vi "CRYDataView Close Panel.vi"(8 "Panel_Idx":i32, 11 "DataView Index":i32) -> (0 "bResult":bool, 2 "bHaveChild":bool, 3 "closed_spliter_idx":i32)   [LabVIEW 2013]
uses:
  CRYNew View Global.vi
panel:
  in  "sp_mdown_hei":i32
  in  "sp_mdown_wid":i32
  in  "sp_mdown_ypos":i32
  in  "sp_mdown_xpos":i32
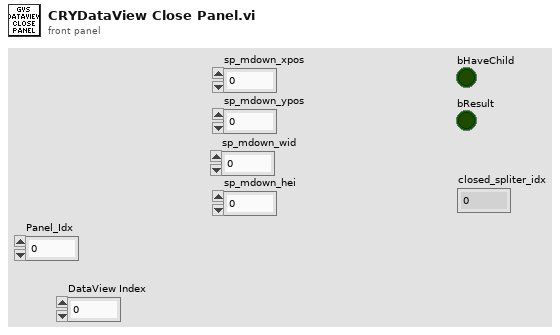
[diagram p1: front panel]
types:
  T1 = typedef "Graph Main Info Cluster.ctl" = cluster{"Selected_BarIdx":i32, "Selected_PanelIdx":i32, "Graph Main VIRef":refnum<vi>, "ToolBarClick":bool, "Spliter Ref Array":refnum<vi>[], "Panel Ref Array":refnum<vi>[], "Spliter_matrix":i32[][], "Panel_matrix":i32[][], "child_spliterIdx_matrix":i32[][], "split_pos_matrix":i32[][], "Title State":bool, "sQueueName":string, "Frame nID":i32, "Graph VIRef Array":cluster{"Graph VIRef":refnum<vi>, "Panel Idx":i32, "Frame VIRef":refnum<vi>, "Icon Ring":i32, "Graph Type":string}[], "View Type":string}
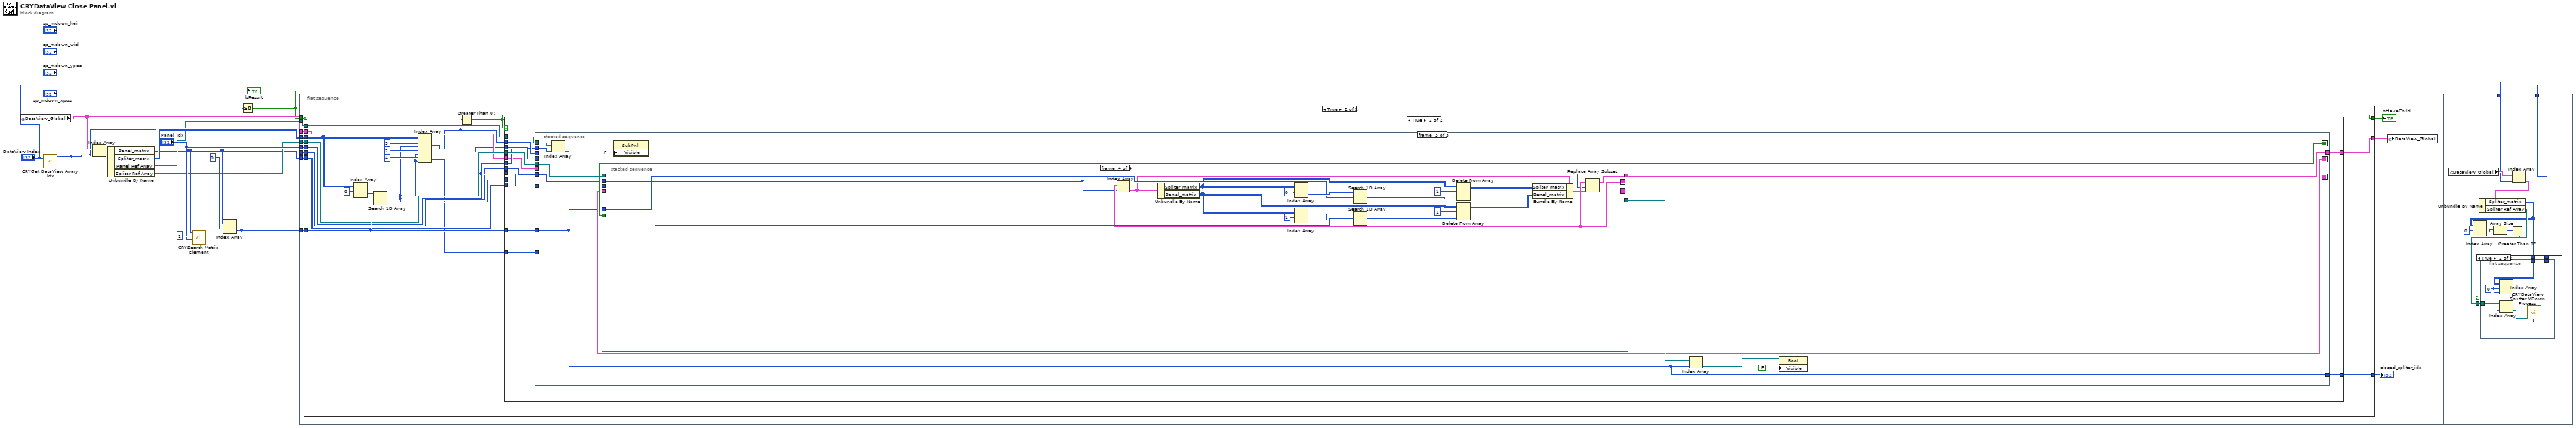
[diagram p0: block diagram]
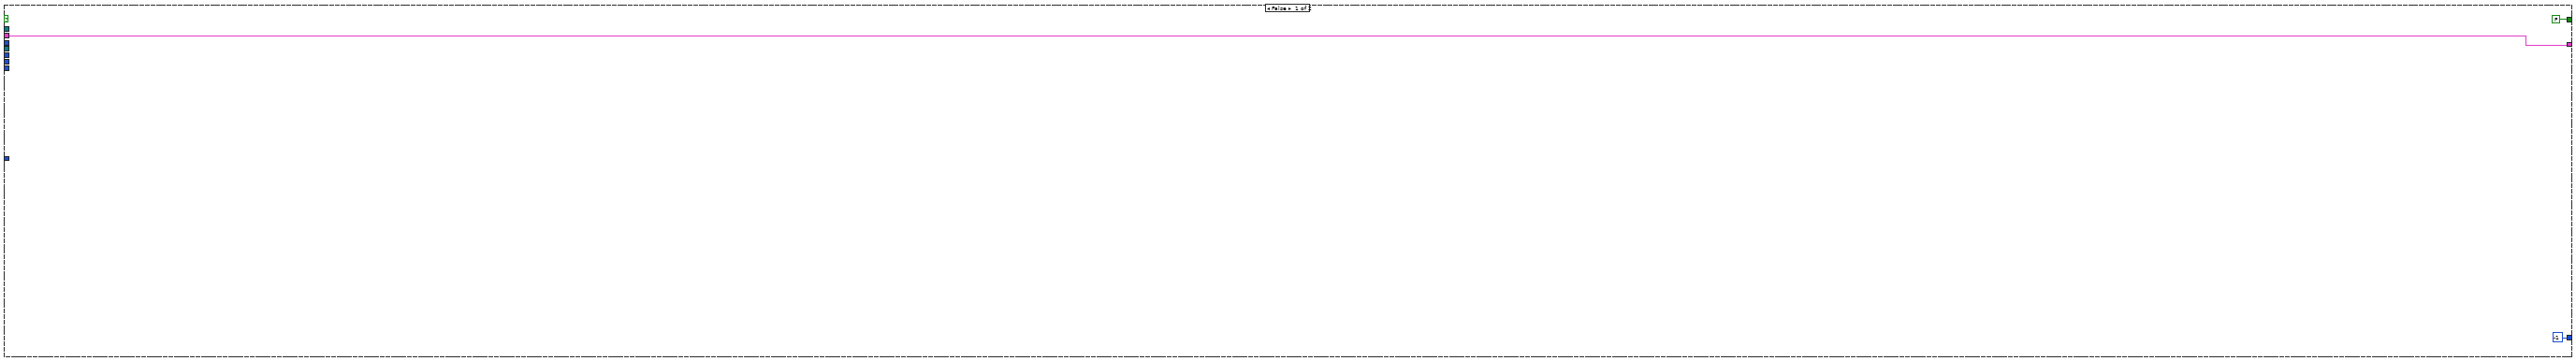
[diagram p2: hidden frame]
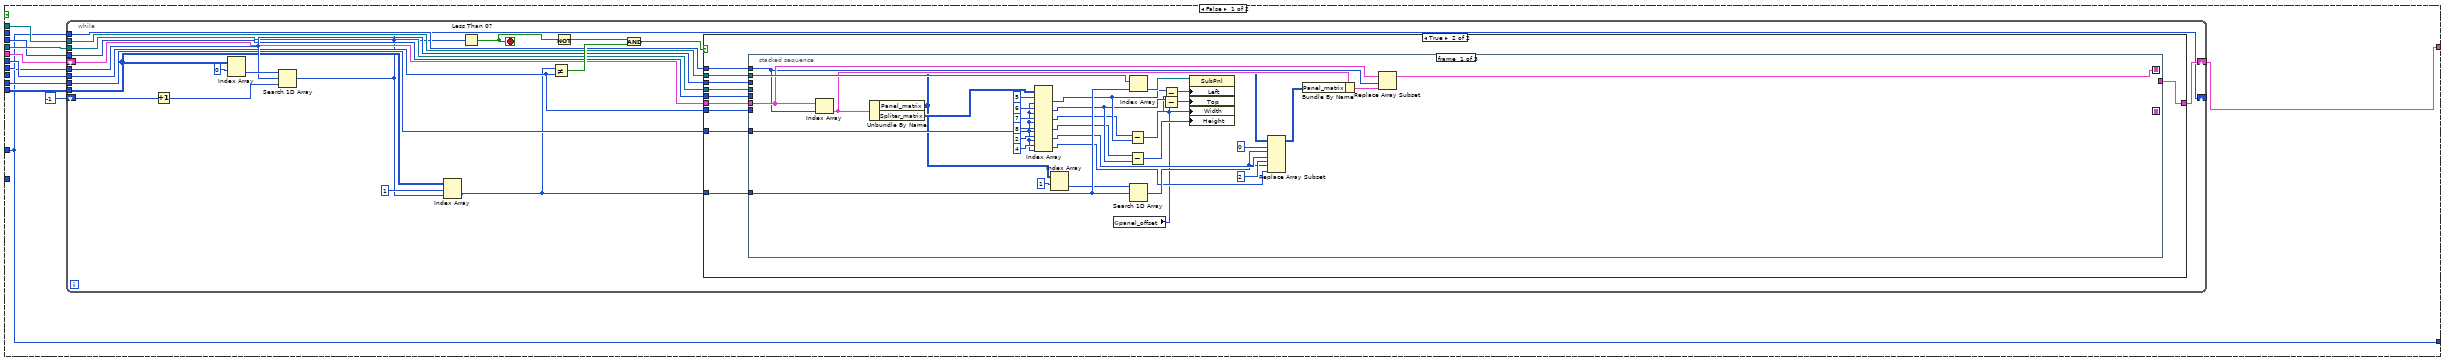
[diagram p3: hidden frame]
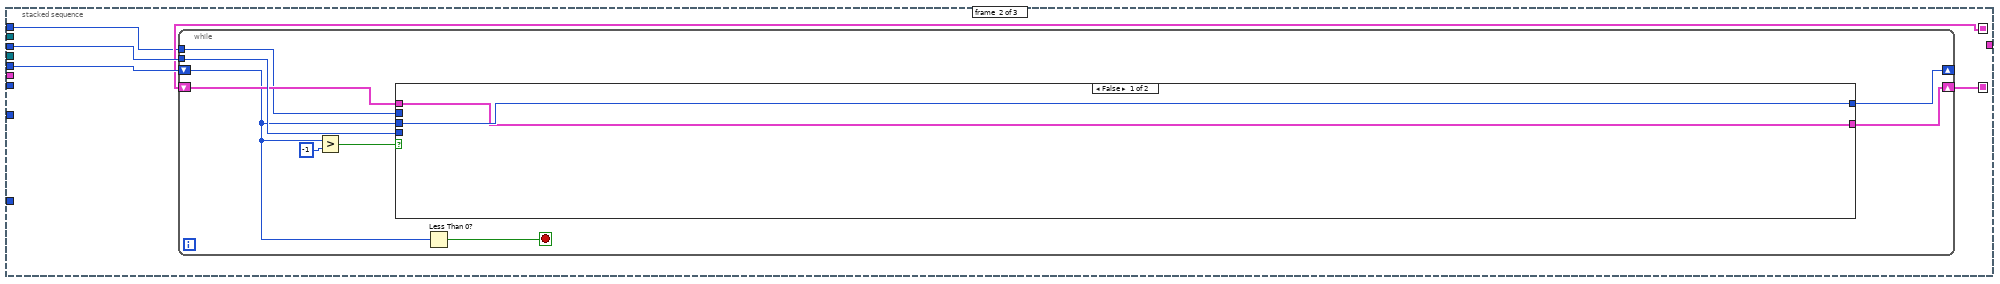
[diagram p5: hidden frame]
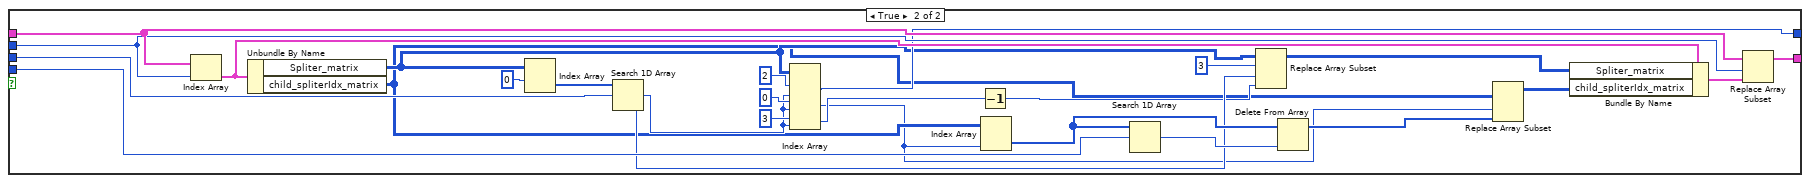
[diagram p6: hidden frame]
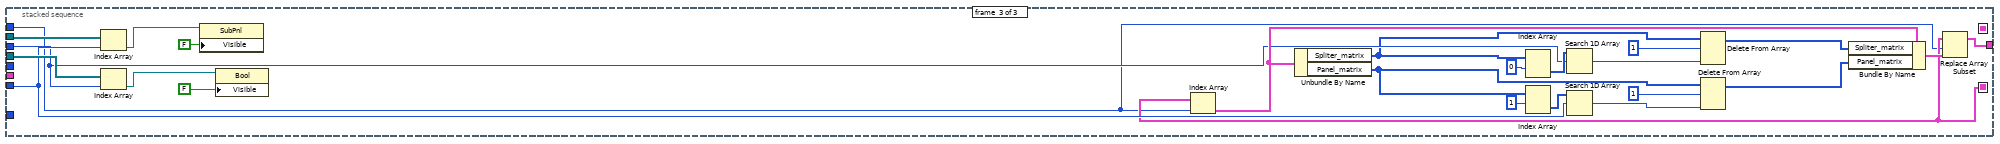
[diagram p7: hidden frame]
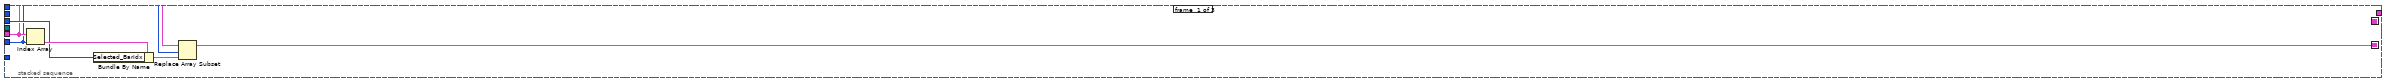
[diagram p8: hidden frame]
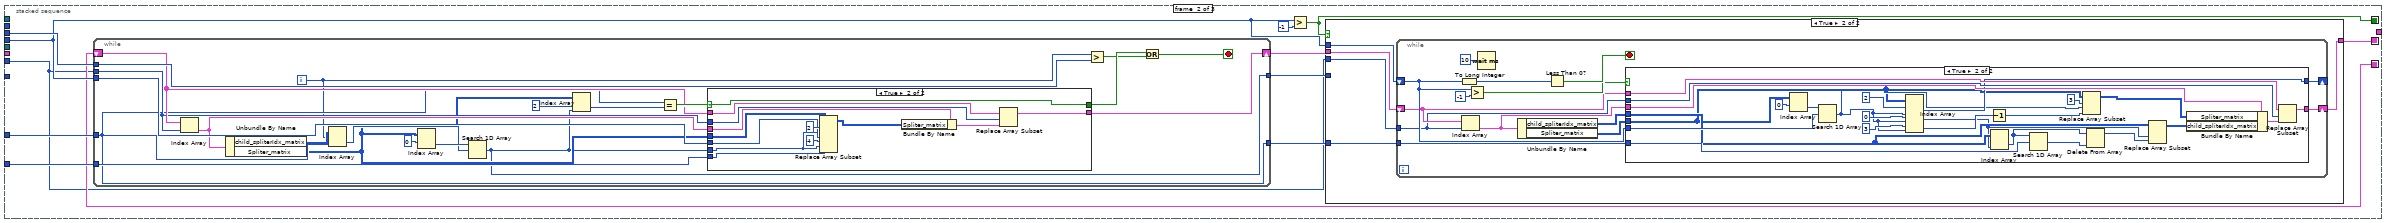
[diagram p9: hidden frame]
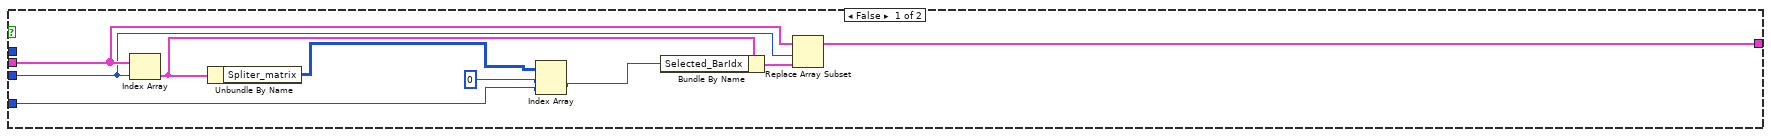
[diagram p10: hidden frame]
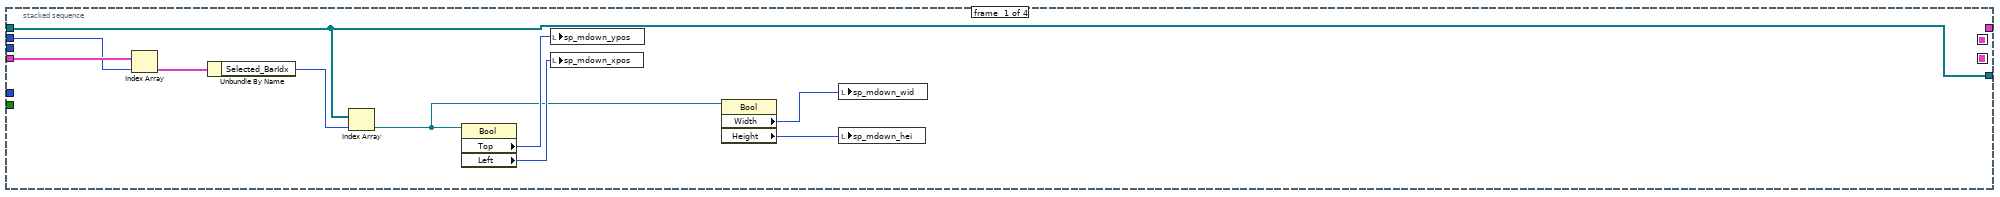
[diagram p13: hidden frame]
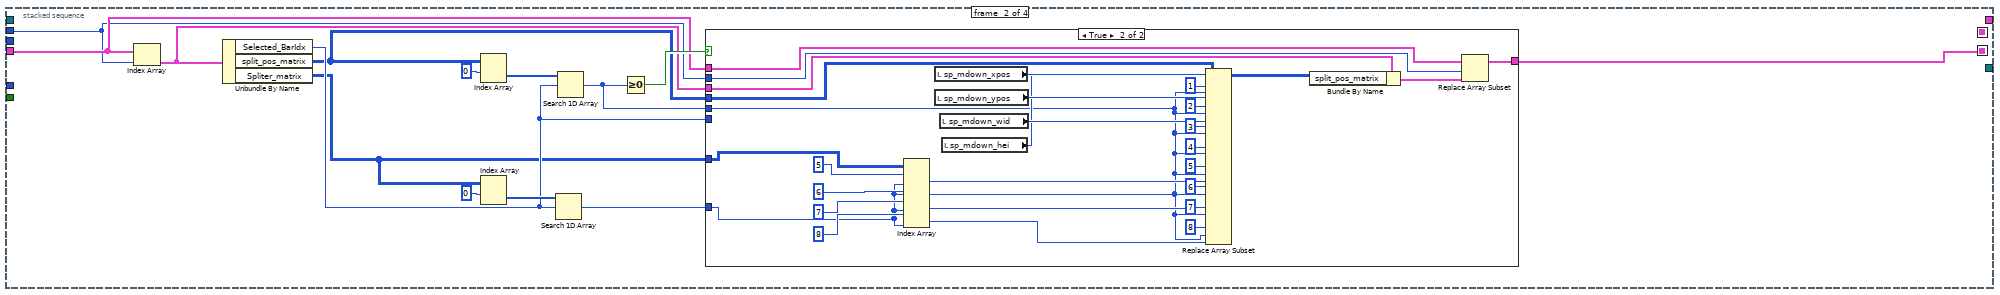
[diagram p14: hidden frame]
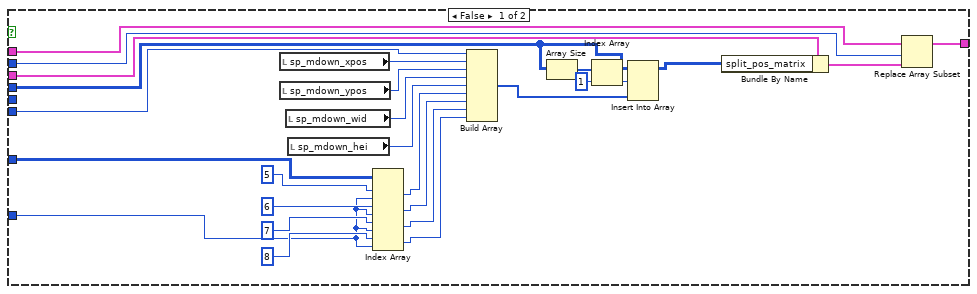
[diagram p15: hidden frame]
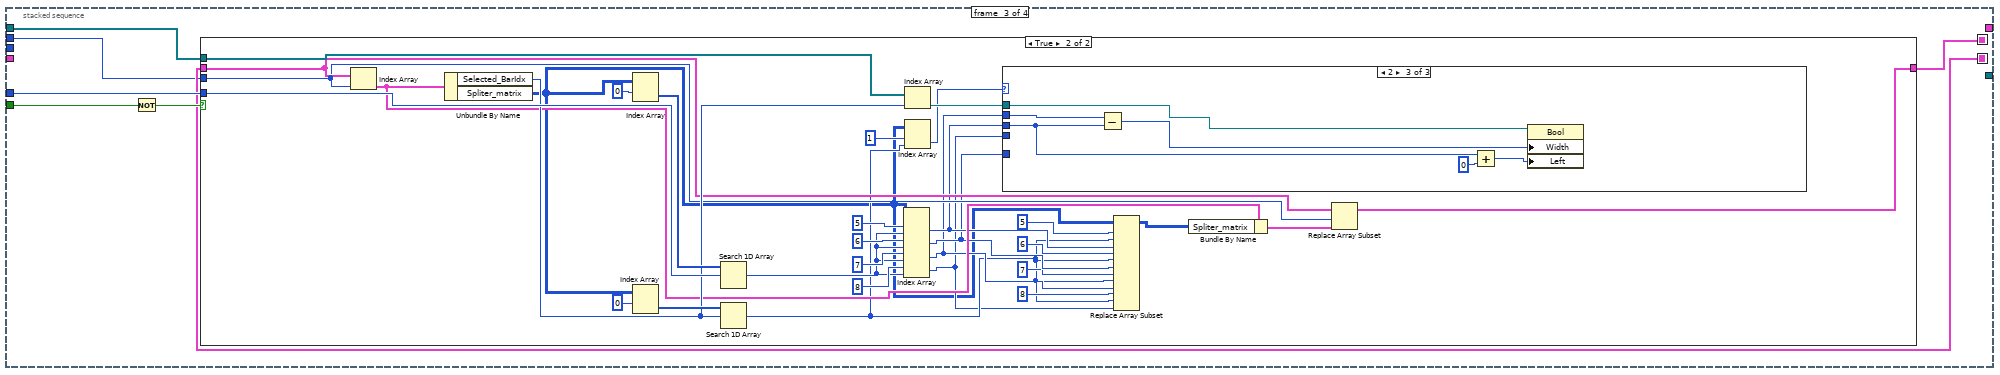
[diagram p16: hidden frame]
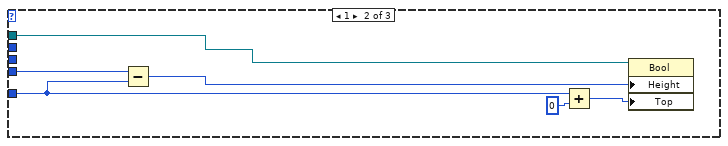
[diagram p19: hidden frame]
diagram:
  n1 = global read "CRYNew View Global.vi" "DataView_Global"() -> (w10:T1[])
  n2 = call "CRYGet DataView Arrary Idx.vi"("DataView Idx In"="DataView Index") -> ("DataView Arrary Idx out"=w2:i32)  [unwired: 10 in]
  n3 = Index Array(array=w10, index=w2) -> (element=w14:T1)
  n4 = Unbundle By Name(w14) -> ("Panel_matrix"=w6:i32[][], "Spliter_matrix"=w12:i32[][], "Panel Ref Array"=w8:refnum<vi>[], "Spliter Ref Array"=w7:refnum<vi>[])
  n5 = call "CRYSearch Matrix Element.vi"("element"="Panel_Idx", "index (row)"=1, "matrix in"=w6) -> ("index of element"=w4:i32)  [unwired: 8 in]
  n6 = Index Array(array=w6, index (row)=0, index (col)=w4) -> (element=w3:i32)
  n7 = Greater Or Equal To 0?(x=w3) -> (x >= 0?=w9:bool)
  "bResult" <- w9
  n8 = flat-sequence {
    tunnel: w12 -> [w26]
    tunnel: w6 -> [w25]
    tunnel: w7 -> [w24]
    tunnel: w8 -> [w23]
    tunnel: w3 -> [w21]
    tunnel: "Panel_Idx" -> [w20]
    tunnel: w10 -> [w19]
    tunnel: w2 -> [w17]
    tunnel: w9 -> [w16]
    tunnel: w2 -> [w479]
    tunnel: "DataView Index" -> [w478]
    frame #0 {
      n9 = case shown="True" w16 {
        tunnel: w21 -> [_ w47]
        tunnel: w24 -> [_ w46]
        tunnel: w23 -> [_ w45]
        tunnel: w20 -> [_ w44]
        tunnel: w26 -> [_ w30]
        tunnel: w25 -> [_ w43]
        tunnel: [w28 w42] -> w18
        tunnel: [FALSE w41] -> w22
        tunnel: w19 -> [w28 w40]
        tunnel: w17 -> [_ w39]
        tunnel: [-1 ("Real Matrix Element") w38] -> w15
        frame False {
        }
        frame True {
          n10 = Index Array(array=w30, index (row)=0) -> (element=w48:i32[])  [unwired: 1 in]
          n11 = Search 1D Array(1D array=w48, element=w47) -> (index of element=w34:i32)  [unwired: 1 in]
          n12 = Index Array(array=w30, index (row) #1=3 ("index (row)"), index (col) #1=w34, index (row) #2=2 ("index (row)"), index (col) #2=w34, index (row) #3=4 ("index (row)"), index (col) #3=w34) -> (element #1=w31:i32, element #2=w33:i32, element #3=w32:i32)
          n13 = Greater Than 0?(x=w31) -> (x > 0?=w41:bool)
          n14 = case shown="True" w41 {
            tunnel: w33 -> [w55 w202]
            tunnel: w47 -> [w50 w203]
            tunnel: w31 -> [_ w204]
            tunnel: w32 -> [_ w198]
            tunnel: w46 -> [w56 w201]
            tunnel: w45 -> [w58 w200]
            tunnel: w44 -> [w59 w199]
            tunnel: w34 -> [w57 _]
            tunnel: w44 -> [_ w197]
            tunnel: w43 -> [w54 _]
            tunnel: [w51 w196] -> w42
            tunnel: w40 -> [w53 w195]
            tunnel: w39 -> [w52 w194]
            tunnel: [w50 w193] -> w38
            frame False {
              n15 = while {
                shift-right: [w62] -> _
                shift-left: -1 -> [w78]
                tunnel: w50 -> [w73]
                tunnel: w59 -> [w69]
                tunnel: w58 -> [w74]
                tunnel: w57 -> [w72]
                tunnel: w55 -> [w71]
                tunnel: w56 -> [w70]
                tunnel: w54 -> [w64]
                tunnel: w52 -> [w66]
                shift-right: [w65] -> w51
                shift-left: w53 -> [w67]
                stop <- w77 stop-if-true
                n16 = Increment(x=w78) -> (x+1=w79:i32)
                n17 = Index Array(array=w64, index (row)=0) -> (element=w80:i32[])  [unwired: 1 in]
                n18 = Search 1D Array(1D array=w80, element=w73, start index (0)=w79) -> (index of element=w62:i32)
                n19 = Index Array(array=w64, index (row)=1, index (col)=w62) -> (element=w61:i32)
                n20 = Less Than 0?(x=w62) -> (x < 0?=w77:bool)
                n21 = Not Equal?(x=w61, y=w69) -> (x != y?=w75:bool)
                n22 = Not(x=w77) -> (.not. x?=w76:bool)
                n23 = And(x=w76, y=w75) -> (x .and. y?=w68:bool)
                n24 = case shown="True" w68 {
                  tunnel: w61 -> [_ w92]
                  tunnel: w74 -> [_ w91]
                  tunnel: w73 -> [_ w90]
                  tunnel: w72 -> [_ w89]
                  tunnel: w71 -> [_ w88]
                  tunnel: w70 -> [_ w87]
                  tunnel: w69 -> [_ w86]
                  tunnel: [w82 w85] -> w65
                  tunnel: w67 -> [w82 w84]
                  tunnel: w66 -> [_ w83]
                  frame False {
                  }
                  frame True {
                    n25 = stacked-sequence {
                      seq-local: [w116 _ _] -> [_ w129 _]
                      seq-local: [_ w128 _] -> [_ _ w173]
                      tunnel: w92 -> [w126 _ _]
                      tunnel: w91 -> [w125 _ w188]
                      tunnel: w90 -> [_ w130 w175]
                      tunnel: w89 -> [w103 _ _]
                      tunnel: w88 -> [_ w131 _]
                      tunnel: w87 -> [_ _ w187]
                      tunnel: w86 -> [_ _ w178]
                      tunnel: [_ _ w174] -> w85
                      tunnel: w84 -> [w117 _ _]
                      tunnel: w83 -> [w115 w127 w172]
                      frame #0 {
                        n26 = Index Array(array=w117, index=w115) -> (element=w118:T1)
                        n27 = Unbundle By Name(w118) -> ("Panel_matrix"=w102:i32[][], "Spliter_matrix"=w114:i32[][])
                        n28 = Index Array(array=w114, index (row) #1=5 ("index (row)"), index (col) #1=w103, index (row) #2=6 ("index (row)"), index (col) #2=w103, index (row) #3=7 ("index (row)"), index (col) #3=w103, index (row) #4=8 ("index (row)"), index (col) #4=w103, index (row) #5=2 ("index (row)"), index (col) #5=w103, index (row) #6=4 ("index (row)"), index (col) #6=w103) -> (element #1=w107:i32, element #2=w106:i32, element #3=w105:i32, element #4=w104:i32, element #5=w100:i32, element #6=w97:i32)
                        n29 = Index Array(array=w102, index (row)=1) -> (element=w120:i32[])  [unwired: 1 in]
                        n30 = global read "CRYNew View Global.vi" "panel_offset"() -> (w93:i32)
                        n31 = Subtract(x=w105, y=w107) -> (x-y=w122:i32)
                        n32 = Subtract(x=w104, y=w106) -> (x-y=w123:i32)
                        n33 = Index Array(array=w125, index=w126) -> (element=w124:refnum<vi>)
                        n34 = Search 1D Array(1D array=w120, element=w126) -> (index of element=w98:i32)  [unwired: 1 in]
                        n35 = Subtract(x=w106, y=w93) -> (x-y=w95:i32)
                        n36 = Subtract(x=w107, y=w93) -> (x-y=w94:i32)
                        n37 = property class="SubPnl"(reference=w124, "Left"=w94, "Top"=w95, "Width"=w122, "Height"=w123) -> ()  [unwired: 1 in, 2 out]
                        n38 = Replace Array Subset(array=w102, new element #1=w100, index (row) #1=0 ("disabled index (row)"), index (col) #1=w98, new element #2=w97, index (row) #2=2 ("disabled index (row)"), index (col) #2=w98) -> (w96:i32[][])
                        n39 = Bundle By Name(cluster=w118, "Panel_matrix"=w96) -> (w119:T1)
                        n40 = Replace Array Subset(array=w117, new element=w119, index=w115) -> (w116:T1[])
                      }
                      frame #1 {
                        n41 = while {
                          shift-right: [w140] -> _
                          shift-left: w131 -> [w132]
                          tunnel: w130 -> [w138]
                          shift-right: [w134] -> w128
                          shift-left: w129 -> [w135]
                          tunnel: w127 -> [w133]
                          stop <- w139 stop-if-true
                          n42 = Greater?(x=w132, y=-1) -> (0:w136:bool)
                          n43 = case shown="False" w136 {
                            tunnel: [w142 w153] -> w140
                            tunnel: w132 -> [w142 w167]
                            tunnel: w138 -> [_ w166]
                            tunnel: w135 -> [w141 w159]
                            tunnel: [w141 w158] -> w134
                            tunnel: w133 -> [_ w157]
                            frame False {
                            }
                            frame True {
                              n44 = Index Array(array=w159, index=w157) -> (element=w160:T1)
                              n45 = Unbundle By Name(w160) -> ("Spliter_matrix"=w147:i32[][], "child_spliterIdx_matrix"=w146:i32[][])
                              n46 = Index Array(array=w147, index (row)=0) -> (element=w164:i32[])  [unwired: 1 in]
                              n47 = Search 1D Array(1D array=w164, element=w167) -> (index of element=w150:i32)  [unwired: 1 in]
                              n48 = Index Array(array=w147, index (row) #1=2 ("index (row)"), index (col) #1=w150, index (row) #2=0 ("index (row)"), index (col) #2=w150, index (row) #3=3 ("index (row)"), index (col) #3=w150) -> (element #1=w153:i32, element #2=w143:i32, element #3=w152:i32)
                              n49 = Decrement(x=w152) -> (x-1=w149:i32)
                              n50 = Index Array(array=w146, index (col)=w143) -> (element=w163:i32[])  [unwired: 1 in]
                              n51 = Search 1D Array(1D array=w163, element=w166) -> (index of element=w162:i32)  [unwired: 1 in]
                              n52 = Replace Array Subset(array=w147, new element=w149, index (row)=3 ("disabled index (row)"), index (col)=w150) -> (w148:i32[][])
                              n53 = Delete From Array(array=w163, index=w162) -> (array with subset deleted=w145:i32[])  [unwired: 1 in, 1 out]
                              n54 = Replace Array Subset(array=w146, new element=w145, index (col)=w143) -> (w144:i32[][])  [unwired: 1 in]
                              n55 = Bundle By Name(cluster=w160, "Spliter_matrix"=w148, "child_spliterIdx_matrix"=w144) -> (w161:T1)
                              n56 = Replace Array Subset(array=w159, new element=w161, index=w157) -> (w158:T1[])
                            }
                          }
                          n57 = Less Than 0?(x=w132) -> (x < 0?=w139:bool)
                        }
                      }
                      frame #2 {
                        n58 = Index Array(array=w188, index=w178) -> (element=w190:refnum<vi>)
                        n59 = Index Array(array=w187, index=w175) -> (element=w192:refnum<vi>)
                        n60 = property class="SubPnl"(reference=w190, "Visible"=FALSE) -> ()  [unwired: 1 in, 2 out]
                        n61 = property class="Bool"(reference=w192, "Visible"=FALSE) -> ()  [unwired: 1 in, 2 out]
                        n62 = Index Array(array=w173, index=w172) -> (element=w176:T1)
                        n63 = Unbundle By Name(w176) -> ("Spliter_matrix"=w171:i32[][], "Panel_matrix"=w170:i32[][])
                        n64 = Index Array(array=w171, index (row)=0) -> (element=w186:i32[])  [unwired: 1 in]
                        n65 = Index Array(array=w170, index (row)=1) -> (element=w179:i32[])  [unwired: 1 in]
                        n66 = Search 1D Array(1D array=w186, element=w175) -> (index of element=w184:i32)  [unwired: 1 in]
                        n67 = Search 1D Array(1D array=w179, element=w178) -> (index of element=w181:i32)  [unwired: 1 in]
                        n68 = Delete From Array(array=w171, length=1, index (col)=w184) -> (array with subset deleted=w169:i32[][])  [unwired: 1 in, 1 out]
                        n69 = Delete From Array(array=w170, length=1, index (col)=w181) -> (array with subset deleted=w168:i32[][])  [unwired: 1 in, 1 out]
                        n70 = Bundle By Name(cluster=w176, "Spliter_matrix"=w169, "Panel_matrix"=w168) -> (w177:T1)
                        n71 = Replace Array Subset(array=w173, new element=w177, index=w172) -> (w174:T1[])
                      }
                    }
                  }
                }
              }
            }
            frame True {
              n72 = stacked-sequence {
                seq-local: [_ w215 _] -> [_ _ w319]
                seq-local: [w206 _ _] -> [_ w214 _]
                seq-local: [_ w213 _] -> [_ _ w316]
                tunnel: w204 -> [_ w222 _]
                tunnel: w203 -> [_ w221 w314]
                tunnel: w202 -> [w208 w218 _]
                tunnel: w201 -> [_ _ w327]
                tunnel: w200 -> [_ _ w323]
                tunnel: w199 -> [_ _ w322]
                tunnel: w198 -> [_ w220 _]
                tunnel: w197 -> [_ _ w318]
                tunnel: [_ _ w317] -> w196
                tunnel: w195 -> [w207 _ _]
                tunnel: w194 -> [w205 w212 w315]
                tunnel: [_ _ w314] -> w193
                frame #0 {
                  n73 = Index Array(array=w207, index=w205) -> (element=w209:T1)
                  n74 = Bundle By Name(cluster=w209, "Selected_BarIdx"=w208) -> (w210:T1)
                  n75 = Replace Array Subset(array=w207, new element=w210, index=w205) -> (w206:T1[])
                }
                frame #1 {
                  n76 = while {
                    tunnel: w221 -> [w284]
                    tunnel: w222 -> [w291]
                    tunnel: w218 -> [w295]
                    tunnel: w220 -> [w290]
                    tunnel: [w284] -> w219
                    tunnel: [w279] -> w216
                    shift-right: [w287] -> w211
                    shift-left: w214 -> [w288]
                    tunnel: w212 -> [w286]
                    i -> [w283]
                    stop <- w292 stop-if-true
                    n77 = Index Array(array=w288, index=w286) -> (element=w289:T1)
                    n78 = Unbundle By Name(w289) -> ("child_spliterIdx_matrix"=w285:i32[][], "Spliter_matrix"=w281:i32[][])
                    n79 = Index Array(array=w285, index (row)=w283, index (col)=w284) -> (element=w282:i32)
                    n80 = Index Array(array=w281, index (row)=0) -> (element=w298:i32[])  [unwired: 1 in]
                    n81 = Search 1D Array(1D array=w298, element=w282) -> (index of element=w279:i32)  [unwired: 1 in]
                    n82 = Index Array(array=w281, index (row)=2, index (col)=w279) -> (element=w278:i32)
                    n83 = Equal?(x=w284, y=w278) -> (x = y?=w296:bool)
                    n84 = case shown="True" w296 {
                      selector: w296 -> [w300 w313]
                      tunnel: w279 -> [_ w301]
                      tunnel: w295 -> [_ w303]
                      tunnel: [w300 w313] -> w294
                      tunnel: w290 -> [_ w304]
                      tunnel: w281 -> [_ w307]
                      tunnel: w289 -> [_ w311]
                      tunnel: w286 -> [_ w310]
                      tunnel: w288 -> [w299 w309]
                      tunnel: [w299 w308] -> w287
                      frame False {
                      }
                      frame True {
                        n85 = Replace Array Subset(array=w307, new element #1=w303, index (row) #1=2 ("disabled index (row)"), index (col) #1=w301, new element #2=w304, index (row) #2=4 ("disabled index (row)"), index (col) #2=w301) -> (w302:i32[][])
                        n86 = Bundle By Name(cluster=w311, "Spliter_matrix"=w302) -> (w312:T1)
                        n87 = Replace Array Subset(array=w309, new element=w312, index=w310) -> (w308:T1[])
                      }
                    }
                    n88 = Greater?(x=w283, y=w291) -> (0:w293:bool)
                    n89 = Or(x=w294, y=w293) -> (x .or. y?=w292:bool)
                  }
                  n90 = Greater?(x=w218, y=-1) -> (0:w215:bool)
                  n91 = case shown="True" w215 {
                    tunnel: w218 -> [_ w236]
                    tunnel: w219 -> [_ w235]
                    tunnel: w216 -> [w224 _]
                    tunnel: w211 -> [w229 w234]
                    tunnel: [w228 w233] -> w213
                    tunnel: w212 -> [w227 w232]
                    frame False {
                      n92 = Index Array(array=w229, index=w227) -> (element=w230:T1)
                      n93 = Unbundle By Name(w230) -> ("Spliter_matrix"=w226:i32[][])
                      n94 = Index Array(array=w226, index (row)=0, index (col)=w224) -> (element=w223:i32)
                      n95 = Bundle By Name(cluster=w230, "Selected_BarIdx"=w223) -> (w231:T1)
                      n96 = Replace Array Subset(array=w229, new element=w231, index=w227) -> (w228:T1[])
                    }
                    frame True {
                      n97 = while {
                        shift-right: [w250] -> _
                        shift-left: w236 -> [w245]
                        tunnel: w235 -> [w247]
                        shift-right: [w238] -> w233
                        shift-left: w234 -> [w239]
                        tunnel: w232 -> [w237]
                        stop <- w248 stop-if-true
                        n98 = To Long Integer(number=w245) -> (32bit integer=w249:i32)
                        n99 = Index Array(array=w239, index=w237) -> (element=w240:T1)
                        n100 = Greater?(x=w245, y=-1) -> (0:w243:bool)
                        n101 = Wait (ms)(milliseconds to wait=u32 10) -> ()  [unwired: 1 out]
                        n102 = Unbundle By Name(w240) -> ("child_spliterIdx_matrix"=w242:i32[][], "Spliter_matrix"=w241:i32[][])
                        n103 = Less Than 0?(x=w249) -> (x < 0?=w248:bool)
                        n104 = case shown="True" w243 {
                          tunnel: [w252 w263] -> w250
                          tunnel: w245 -> [w252 w277]
                          tunnel: w247 -> [_ w276]
                          tunnel: w241 -> [_ w253]
                          tunnel: w242 -> [_ w257]
                          tunnel: w240 -> [_ w270]
                          tunnel: w237 -> [_ w269]
                          tunnel: w239 -> [w251 w268]
                          tunnel: [w251 w267] -> w238
                          frame False {
                          }
                          frame True {
                            n105 = Index Array(array=w253, index (row)=0) -> (element=w274:i32[])  [unwired: 1 in]
                            n106 = Search 1D Array(1D array=w274, element=w277) -> (index of element=w260:i32)  [unwired: 1 in]
                            n107 = Index Array(array=w253, index (row) #1=2 ("index (row)"), index (col) #1=w260, index (row) #2=0 ("index (row)"), index (col) #2=w260, index (row) #3=3 ("index (row)"), index (col) #3=w260) -> (element #1=w263:i32, element #2=w256:i32, element #3=w262:i32)
                            n108 = Decrement(x=w262) -> (x-1=w259:i32)
                            n109 = Index Array(array=w257, index (col)=w256) -> (element=w273:i32[])  [unwired: 1 in]
                            n110 = Search 1D Array(1D array=w273, element=w276) -> (index of element=w272:i32)  [unwired: 1 in]
                            n111 = Replace Array Subset(array=w253, new element=w259, index (row)=3 ("disabled index (row)"), index (col)=w260) -> (w258:i32[][])
                            n112 = Delete From Array(array=w273, index=w272) -> (array with subset deleted=w255:i32[])  [unwired: 1 in, 1 out]
                            n113 = Replace Array Subset(array=w257, new element=w255, index (col)=w256) -> (w254:i32[][])  [unwired: 1 in]
                            n114 = Bundle By Name(cluster=w270, "Spliter_matrix"=w258, "child_spliterIdx_matrix"=w254) -> (w271:T1)
                            n115 = Replace Array Subset(array=w268, new element=w271, index=w269) -> (w267:T1[])
                          }
                        }
                      }
                    }
                  }
                }
                frame #2 {
                  n116 = Index Array(array=w323, index=w322) -> (element=w321:refnum<vi>)
                  n117 = stacked-sequence {
                    seq-local: [_ w341 _ _] -> [_ _ w410 _]
                    seq-local: [_ _ w409 _] -> [_ _ _ w464]
                    tunnel: w327 -> [w333 _ w411 _]
                    tunnel: [w333 _ _ _] -> w326
                    tunnel: w314 -> [_ _ w414 w475]
                    tunnel: w319 -> [_ _ w413 _]
                    tunnel: w318 -> [_ _ _ w468]
                    tunnel: [_ _ _ w465] -> w317
                    tunnel: w316 -> [w330 w342 _ _]
                    tunnel: w315 -> [w329 w340 w408 w463]
                    frame #0 {
                      n118 = Index Array(array=w330, index=w329) -> (element=w332:T1)
                      n119 = Unbundle By Name(w332) -> ("Selected_BarIdx"=w331:i32)
                      n120 = Index Array(array=w333, index=w331) -> (element=w328:refnum<vi>)
                      n121 = property class="Bool"(reference=w328) -> ("Top"=w337:i32, "Left"=w336:i32)  [unwired: 1 in, 2 out]
                      n122 = local write "sp_mdown_ypos"(w337) -> ()
                      n123 = local write "sp_mdown_xpos"(w336) -> ()
                      n124 = property class="Bool"(reference=w328) -> ("Width"=w335:u32, "Height"=w334:u32)  [unwired: 1 in, 2 out]
                      n125 = local write "sp_mdown_wid"(w335) -> ()
                      n126 = local write "sp_mdown_hei"(w334) -> ()
                    }
                    frame #1 {
                      n127 = Index Array(array=w342, index=w340) -> (element=w343:T1)
                      n128 = Unbundle By Name(w343) -> ("Selected_BarIdx"=w344:i32, "split_pos_matrix"=w339:i32[][], "Spliter_matrix"=w338:i32[][])
                      n129 = Index Array(array=w339, index (row)=0) -> (element=w349:i32[])  [unwired: 1 in]
                      n130 = Index Array(array=w338, index (row)=0) -> (element=w346:i32[])  [unwired: 1 in]
                      n131 = Search 1D Array(1D array=w346, element=w344) -> (index of element=w345:i32)  [unwired: 1 in]
                      n132 = Search 1D Array(1D array=w349, element=w344) -> (index of element=w350:i32)  [unwired: 1 in]
                      n133 = Greater Or Equal To 0?(x=w350) -> (x >= 0?=w351:bool)
                      n134 = case shown="True" w351 {
                        tunnel: w350 -> [_ w378]
                        tunnel: w344 -> [w373 _]
                        tunnel: w345 -> [w362 w397]
                        tunnel: w338 -> [w367 w398]
                        tunnel: w339 -> [w354 w396]
                        tunnel: w343 -> [w371 w406]
                        tunnel: w340 -> [w370 w405]
                        tunnel: w342 -> [w369 w404]
                        tunnel: [w368 w403] -> w341
                        frame False {
                          n135 = local read "sp_mdown_xpos"() -> (w374:i32)
                          n136 = local read "sp_mdown_ypos"() -> (w375:i32)
                          n137 = local read "sp_mdown_wid"() -> (w376:i32)
                          n138 = local read "sp_mdown_hei"() -> (w377:i32)
                          n139 = Index Array(array=w367, index (row) #1=5 ("index (row)"), index (col) #1=w362, index (row) #2=6 ("index (row)"), index (col) #2=w362, index (row) #3=7 ("index (row)"), index (col) #3=w362, index (row) #4=8 ("index (row)"), index (col) #4=w362) -> (element #1=w361:i32, element #2=w360:i32, element #3=w359:i32, element #4=w358:i32)
                          n140 = Build Array(w373, w374, w375, w376, w377, w361, w360, w359, w358) -> (w353:i32[])
                          n141 = Array Size(array=w354) -> (size(s)=w357:i32[])
                          n142 = Index Array(array=w357, index=1) -> (element=w355:i32)
                          n143 = Insert Into Array(array=w354, index (col)=w355, new element=w353) -> (w352:i32[][])  [unwired: 1 in]
                          n144 = Bundle By Name(cluster=w371, "split_pos_matrix"=w352) -> (w372:T1)
                          n145 = Replace Array Subset(array=w369, new element=w372, index=w370) -> (w368:T1[])
                        }
                        frame True {
                          n146 = Index Array(array=w398, index (row) #1=5 ("index (row)"), index (col) #1=w397, index (row) #2=6 ("index (row)"), index (col) #2=w397, index (row) #3=7 ("index (row)"), index (col) #3=w397, index (row) #4=8 ("index (row)"), index (col) #4=w397) -> (element #1=w382:i32, element #2=w381:i32, element #3=w380:i32, element #4=w379:i32)
                          n147 = local read "sp_mdown_xpos"() -> (w386:i32)
                          n148 = local read "sp_mdown_ypos"() -> (w385:i32)
                          n149 = local read "sp_mdown_wid"() -> (w384:i32)
                          n150 = local read "sp_mdown_hei"() -> (w383:i32)
                          n151 = Replace Array Subset(array=w396, new element #1=w386, index (row) #1=1 ("disabled index (row)"), index (col) #1=w378, new element #2=w385, index (row) #2=2 ("disabled index (row)"), index (col) #2=w378, new element #3=w384, index (row) #3=3 ("disabled index (row)"), index (col) #3=w378, new element #4=w383, index (row) #4=4 ("disabled index (row)"), index (col) #4=w378, new element #5=w382, index (row) #5=5 ("disabled index (row)"), index (col) #5=w378, new element #6=w381, index (row) #6=6 ("disabled index (row)"), index (col) #6=w378, new element #7=w380, index (row) #7=7 ("disabled index (row)"), index (col) #7=w378, new element #8=w379, index (row) #8=8 ("disabled index (row)"), index (col) #8=w378) -> (w387:i32[][])
                          n152 = Bundle By Name(cluster=w406, "split_pos_matrix"=w387) -> (w407:T1)
                          n153 = Replace Array Subset(array=w404, new element=w407, index=w405) -> (w403:T1[])
                        }
                      }
                    }
                    frame #2 {
                      n154 = Not(x=w413) -> (.not. x?=w412:bool)
                      n155 = case shown="True" w412 {
                        tunnel: w414 -> [_ w445]
                        tunnel: w411 -> [_ w441]
                        tunnel: w410 -> [w415 w436]
                        tunnel: [w415 w435] -> w409
                        tunnel: w408 -> [_ w434]
                        frame False {
                        }
                        frame True {
                          n156 = Index Array(array=w436, index=w434) -> (element=w438:T1)
                          n157 = Unbundle By Name(w438) -> ("Selected_BarIdx"=w439:i32, "Spliter_matrix"=w416:i32[][])
                          n158 = Index Array(array=w416, index (row)=0) -> (element=w446:i32[])  [unwired: 1 in]
                          n159 = Index Array(array=w416, index (row)=0) -> (element=w443:i32[])  [unwired: 1 in]
                          n160 = Search 1D Array(1D array=w446, element=w445) -> (index of element=w427:i32)  [unwired: 1 in]
                          n161 = Search 1D Array(1D array=w443, element=w439) -> (index of element=w418:i32)  [unwired: 1 in]
                          n162 = Index Array(array=w416, index (row) #1=5 ("index (row)"), index (col) #1=w427, index (row) #2=6 ("index (row)"), index (col) #2=w427, index (row) #3=7 ("index (row)"), index (col) #3=w427, index (row) #4=8 ("index (row)"), index (col) #4=w427) -> (element #1=w424:i32, element #2=w422:i32, element #3=w420:i32, element #4=w417:i32)
                          n163 = Index Array(array=w441, index=w439) -> (element=w440:refnum<vi>)
                          n164 = Index Array(array=w416, index (row)=1, index (col)=w418) -> (element=w432:i32)
                          n165 = case shown="2" w432 {
                            tunnel: w440 -> [_ w447 w453]
                            tunnel: w417 -> [_ w452 _]
                            tunnel: w422 -> [_ w450 _]
                            tunnel: w420 -> [_ _ w458]
                            tunnel: w424 -> [_ _ w455]
                            frame 0, Default {
                            }
                            frame 1 {
                              n166 = Subtract(x=w452, y=w450) -> (x-y=w451:i32)
                              n167 = Add(x=w450, y=0) -> (x+y=w448:i32)
                              n168 = property class="Bool"(reference=w447, "Height"=w451, "Top"=w448) -> ()  [unwired: 1 in, 2 out]
                            }
                            frame 2 {
                              n169 = Subtract(x=w458, y=w455) -> (x-y=w457:i32)
                              n170 = Add(x=w455, y=0) -> (x+y=w454:i32)
                              n171 = property class="Bool"(reference=w453, "Width"=w457, "Left"=w454) -> ()  [unwired: 1 in, 2 out]
                            }
                          }
                          n172 = Replace Array Subset(array=w416, new element #1=w424, index (row) #1=5 ("disabled index (row)"), index (col) #1=w418, new element #2=w422, index (row) #2=6 ("disabled index (row)"), index (col) #2=w418, new element #3=w420, index (row) #3=7 ("disabled index (row)"), index (col) #3=w418, new element #4=w417, index (row) #4=8 ("disabled index (row)"), index (col) #4=w418) -> (w426:i32[][])
                          n173 = Bundle By Name(cluster=w438, "Spliter_matrix"=w426) -> (w437:T1)
                          n174 = Replace Array Subset(array=w436, new element=w437, index=w434) -> (w435:T1[])
                        }
                      }
                    }
                    frame #3 {
                      n175 = Index Array(array=w464, index=w463) -> (element=w467:T1)
                      n176 = Unbundle By Name(w467) -> ("Spliter_matrix"=w461:i32[][], "Panel_matrix"=w462:i32[][])
                      n177 = Index Array(array=w461, index (row)=0) -> (element=w477:i32[])  [unwired: 1 in]
                      n178 = Index Array(array=w462, index (row)=1) -> (element=w469:i32[])  [unwired: 1 in]
                      n179 = Search 1D Array(1D array=w477, element=w475) -> (index of element=w474:i32)  [unwired: 1 in]
                      n180 = Search 1D Array(1D array=w469, element=w468) -> (index of element=w471:i32)  [unwired: 1 in]
                      n181 = Delete From Array(array=w461, length=1, index (col)=w474) -> (array with subset deleted=w460:i32[][])  [unwired: 1 in, 1 out]
                      n182 = Delete From Array(array=w462, length=1, index (col)=w471) -> (array with subset deleted=w459:i32[][])  [unwired: 1 in, 1 out]
                      n183 = Bundle By Name(cluster=w467, "Spliter_matrix"=w460, "Panel_matrix"=w459) -> (w466:T1)
                      n184 = Replace Array Subset(array=w464, new element=w466, index=w463) -> (w465:T1[])
                    }
                  }
                  n185 = property class="SubPnl"(reference=w321, "Visible"=FALSE) -> ()  [unwired: 1 in, 2 out]
                  n186 = Index Array(array=w326, index=w314) -> (element=w325:refnum<vi>)
                  n187 = property class="Bool"(reference=w325, "Visible"=FALSE) -> ()  [unwired: 1 in, 2 out]
                }
              }
            }
          }
        }
      }
      "bHaveChild" <- w22
      "closed_spliter_idx" <- w15
      n188 = global write "CRYNew View Global.vi" "DataView_Global"(w18) -> ()
    }
    frame #1 {
      n189 = global read "CRYNew View Global.vi" "DataView_Global"() -> (w487:T1[])
      n190 = Index Array(array=w487, index=w479) -> (element=w486:T1)
      n191 = Unbundle By Name(w486) -> ("Spliter_matrix"=w484:i32[][], "Spliter Ref Array"=w485:refnum<vi>[])
      n192 = Index Array(array=w484, index (row)=0) -> (element=w482:i32[])  [unwired: 1 in]
      n193 = Array Size(array=w482) -> (size(s)=w481:i32)
      n194 = Greater Than 0?(x=w481) -> (x > 0?=w480:bool)
      n195 = case shown="True" w480 {
        tunnel: w485 -> [_ w490]
        tunnel: w484 -> [_ w489]
        tunnel: w478 -> [_ w488]
        frame False {
        }
        frame True {
          n196 = flat-sequence {
            tunnel: w490 -> [w496]
            tunnel: w489 -> [w494]
            tunnel: w488 -> [w491]
            frame #0 {
              w493 = 0 ("index (row)")
              n197 = Index Array(array=w494, index (row)=w493, index (col)=w493) -> (element=w492:i32)
              n198 = Index Array(array=w496, index=w492) -> (element=w495:refnum<vi>)
              n199 = call "CRYDataView Splitter MDown Process.vi"("DataView Index"=w491, "Selected Spliter Ref"=w495) -> ()  [unwired: 9 in, 1 out]
            }
          }
        }
      }
    }
  }
